vi "Cartesian_Experiment.vi"() -> ()   [LabVIEW 2016]
uses:
  <vilib>/gmath/NI_Gmath.lvlib
panel:
  out "Waveform Graph":dbl[][](graph)
  out "Action VIs":path[](array[path])=[path "C:/user/patrick/control_vi/Action_SubVIs/Set_B.vi", path "C:/user/patrick/control_vi/Action_SubVIs/Set_T.vi", path "C:/user/patrick/control_vi/Action_SubVIs/Set_Vsg1.vi", path "C:/user/patrick/control_vi/Action_SubVIs/Set_Vsg2.vi"]
  in  "Number of switch settings":i32
  in  "Tab Control":T1(tab)=enum."File Settings"
  in  "Scan Array (Slow to Fast: priority = 0 to N)":T2(array[cluster])=[{"Ramp Cluster"={"Max"=0.0, "Min"=0.0, "step size"=0.004, "cycles (1,2,...)"=0, "phase (deg)"=0.0, "function (ramp)"=enum."Ramp"}, "Priority"=0, "Action"=0, "Action 2"=0}, {"Ramp Cluster"={"Max"=0.15, "Min"=-0.08, "step size"=0.01, "cycles (1,2,...)"=0, "phase (deg)"=0.0, "function (ramp)"=enum."Ramp"}, "Priority"=2, "Action"=0, "Action 2"=0}, {"Ramp Cluster"={"Max"=0.15, "Min"=-0.15, "step size"=0.001, "cycles (1,2,...)"=0, "phase (deg)"=0.001, "function (ramp)"=enum."Ramp"}, "Priority"=1, "Action"=0, "Action 2"=0}] {"Action 2" items=["single value", "ramp", "vector ramp", "other..."]; "Action" items=["Set_B", "Set_T", "Set_Vsg1", "Set_Vsg2"]; "Ramp Cluster"."phase (deg)" format="%#.4p"; "Ramp Cluster"."cycles (1,2,...)" min=1; "Ramp Cluster"."step size" format="%#.4p"; "Ramp Cluster"."Min" format="%#_6p"; "Ramp Cluster"."Max" format="%#_6p"}
  in  "stop":bool
  in  "AVS_CalFolder":path=path "E:/Dropbox/Labview/LC Software/All Calibrations" caption="Action subVIs files path"
  in  "read T?":bool
  # "Ramp function: Min=START, Max=END\n\nOther functions: \nMax > Min, change phase to control starting value"
  # "Ao1 has a large offset (600mV), an offset it is hard wired to Vsg2"
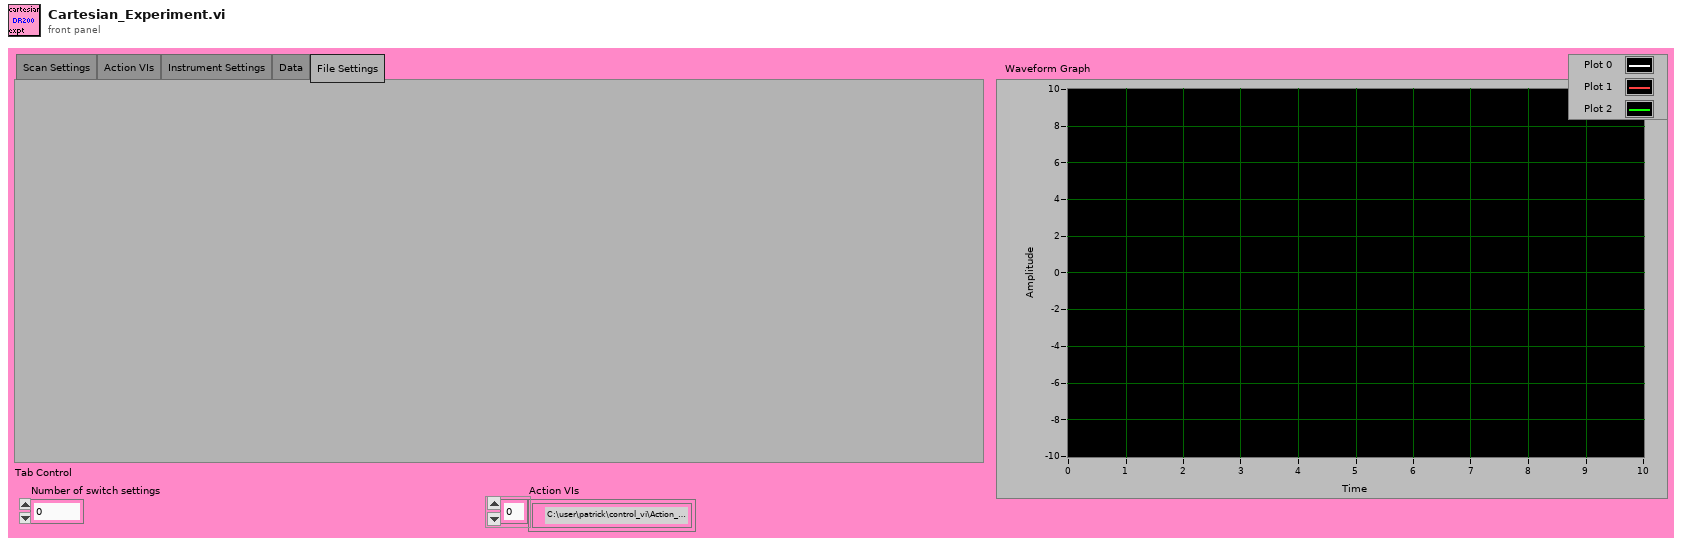
[diagram p1: front panel]
types:
  T1 = enum32{"Scan Settings", "Action VIs", "Instrument Settings", "Data", "File Settings"}
  T2 = cluster{"Ramp Cluster":cluster{"Max":dbl, "Min":dbl, "step size":dbl, "cycles (1,2,...)":i32, "phase (deg)":dbl, "function (ramp)":enum16{"Ramp", "Triangle", "Sine"}}, "Priority":i32, "Action":u16, "Action 2":u16}[]
  T3 = cluster{"Ramp Cluster":cluster{"Max":dbl, "Min":dbl, "step size":dbl, "cycles (1,2,...)":i32, "phase (deg)":dbl, "function (ramp)":enum16{"Ramp", "Triangle", "Sine"}}, "Priority":i32, "Action":u16, "Action 2":u16}
  T4 = enum16{"set T", "set B", "set Vsg1", "set Vsg2", "set lockin DC offset", "Switch"}
  T5 = cluster{"Max":dbl, "Min":dbl, "step size":dbl, "cycles (1,2,...)":i32, "phase (deg)":dbl, "function (ramp)":enum16{"Ramp", "Triangle", "Sine"}}
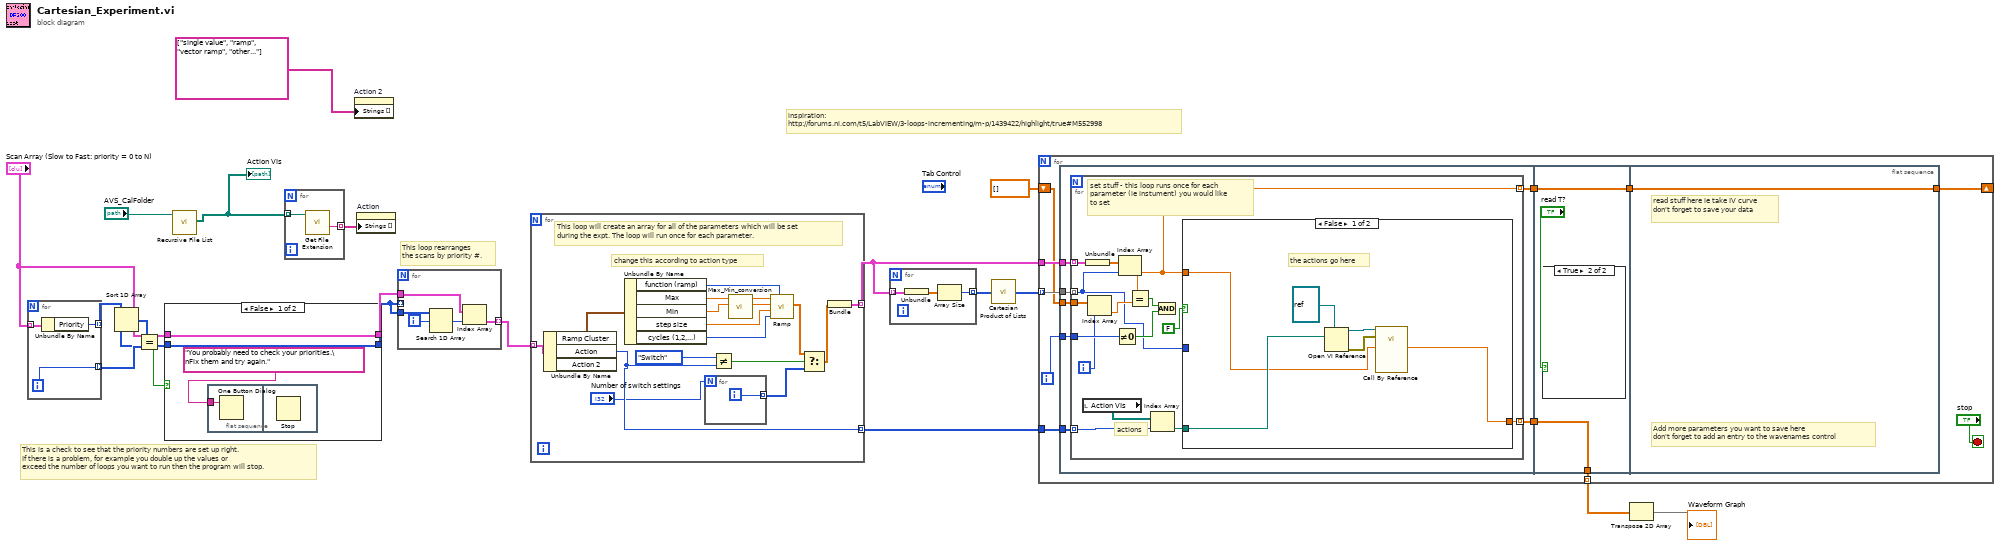
[diagram p0: block diagram]
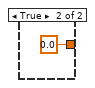
[diagram p2: hidden frame]
diagram:
  # "This loop rearranges\nthe scans by priority #."
  # "This is a check to see that the priority numbers are set up right. \nIf there is a problem, for example you double up the values or \nexceed the number of loops you want to run then the program will stop."
  # "inspiration:\nhttp://forums.ni.com/t5/LabVIEW/3-loops-incrementing/m-p/1439422/highlight/true#M552998"
  n1 = for {
    tunnel: "Scan Array (Slow to Fast: priority = 0 to N)" -> [w22] mode=indexing
    tunnel: [w21] -> w11 mode=indexing
    tunnel: [w20] -> w15 mode=indexing
    i -> [w20]
    n2 = Unbundle By Name(w22) -> ("Priority"=w21:i32)
  }
  n3 = Sort 1D Array(array=w11) -> (sorted array=w16:i32[])
  n4 = Equal?(x=w16, y=w15) -> (x = y?=w14:bool)
  n5 = case shown="False" w14 {
    tunnel: [w24 w28] -> w13
    tunnel: "Scan Array (Slow to Fast: priority = 0 to N)" -> [w24 w28]
    tunnel: [w25 w27] -> w10
    tunnel: w11 -> [w25 w27]
    frame False {
      n6 = flat-sequence {
        tunnel: "You probably need to check your priorities.\nFix them and try again." ("message") -> [w26]
        frame #0 {
          n7 = One Button Dialog(message=w26) -> ()  [unwired: 1 in, 1 out]
        }
        frame #1 {
          n8 = Stop() -> ()  [unwired: 1 in]
        }
      }
    }
    frame True {
    }
  }
  n9 = call <vilib>:"Recursive File List.vi"("Folder Path"="AVS_CalFolder") -> ("All Files in Dir"=w4:path[])  [unwired: 6 in, 4 out]
  "Action VIs" <- w4
  n10 = for {
    tunnel: w4 -> [w30] mode=indexing
    tunnel: [w29] -> w5 mode=indexing
    n11 = call <vilib>:"Get File Extension.vi"("file"=w30) -> ("filename without extension"=w29:string)  [unwired: 6 in, 4 out]
  }
  n12 = property on="Action 2" class="Ring (strict)"("Strings []"=string[] ["single value", "ramp", "vector ramp", "other..."]) -> ()  [unwired: 2 in, 2 out]
  n13 = property on="Action" class="Ring (strict)"("Strings []"=w5) -> ()  [unwired: 2 in, 2 out]
  n14 = for {
    tunnel: w13 -> [w35]
    tunnel: w10 -> [_] mode=indexing
    tunnel: [w34] -> w17 mode=indexing
    tunnel: w10 -> [w33]
    i -> [w32]
    n15 = Search 1D Array(1D array=w33, element=w32) -> (index of element=w31:i32)  [unwired: 1 in]
    n16 = Index Array(array=w35, index=w31) -> (element=w34:T3)
  }
  n17 = for {
    tunnel: [w51] -> w18 mode=indexing
    tunnel: w17 -> [w52] mode=indexing
    tunnel: [w41] -> w19 mode=indexing
    # "change this according to action type"
    # "This loop will create an array for all of the parameters which will be set\nduring the expt. The loop will run once for each parameter."
    n18 = Unbundle By Name(w52) -> ("Ramp Cluster"=w49:T5, "Action"=w41:u16)  [unwired: 1 out]
    n19 = Unbundle By Name(w49) -> ("function (ramp)"=w48:enum16{"Ramp", "Triangle", "Sine"}, "Max"=w47:dbl, "Min"=w46:dbl, "step size"=w44:dbl, "cycles (1,2,...)"=w43:i32)
    n20 = for {
      N: "Number of switch settings" -> [_]
      tunnel: [w53] -> w42 mode=indexing
      i -> [w53]
    }
    n21 = Not Equal?(x=T4."Switch" ("Action"), y=w41) -> (x != y?=w39:bool)
    n22 = call "Max_Min_conversion.vi"("Min"=w46, "Max"=w47) -> ("offset"=w45:dbl, "Amplitude"=w50:dbl)  [unwired: 8 in]
    n23 = call "Ramp.vi"("function (ramp)"=w48, "cycles (1,2,...)"=w43, "step size"=w44, "offset"=w45, "amplitude"=w50) -> ("Waveform Graph"=w38:dbl[])  [unwired: 4 in, 2 out]
    n24 = Select(t=w38, s=w39, f=w42) -> (s? t:f=w37:dbl[])
    n25 = Bundle("Waveform Graph"=w37) -> (w51:cluster{"Waveform Graph":dbl[]})  [unwired: 1 in]
  }
  n26 = for {
    tunnel: w18 -> [w56] mode=indexing
    tunnel: [w54] -> w9 mode=indexing
    n27 = Unbundle(w56) -> ("Waveform Graph"=w55:dbl[])
    n28 = Array Size(array=w55) -> (size(s)=w54:i32)
  }
  n29 = call <vilib>:"Cartesian Product of Lists.vi"("Number of Elements in Each List"=w9) -> ("Cartesian Product of Lists"=w7:i32[][])
  n30 = for {
    tunnel: w7 -> [w67] mode=indexing
    tunnel: w18 -> [w66]
    tunnel: w19 -> [w65]
    shift-right: [w64] -> _
    shift-left: dbl[] [] -> [w63]
    tunnel: [w57] -> w3 mode=indexing
    i -> [w59]
    stop <- "stop" stop-if-true
    n31 = flat-sequence {
      tunnel: w67 -> [w74]
      tunnel: w66 -> [w73]
      tunnel: w65 -> [w72]
      tunnel: w63 -> [w70]
      tunnel: w59 -> [w69]
      tunnel: [w71] -> w62
      tunnel: [w68] -> w58
      tunnel: w62 -> [w99]
      tunnel: [w99] -> w61
      tunnel: w58 -> [w97]
      tunnel: [w97] -> w57
      tunnel: w61 -> [w100]
      tunnel: [w100] -> w64
      frame #0 {
        n32 = for {
          tunnel: w74 -> [w80] mode=indexing
          tunnel: w73 -> [w89] mode=indexing
          tunnel: w72 -> [w79] mode=indexing
          tunnel: [w87] -> w71 mode=indexing
          tunnel: w70 -> [w84]
          tunnel: w69 -> [w82]
          tunnel: [w76] -> w68 mode=indexing
          i -> [w81]
          # "actions"
          # "set stuff - this loop runs once for each\nparameter (ie instument) you would like\nto set"
          n33 = local read "Action VIs"() -> (w78:path[])
          n34 = Unbundle(w89) -> ("Waveform Graph"=w88:dbl[])
          n35 = Index Array(array=w84, index=w81) -> (element=w83:dbl)
          n36 = Not Equal To 0?(x=w82) -> (x != 0?=w86:bool)
          n37 = Index Array(array=w88, index=w80) -> (element=w87:dbl)
          n38 = Equal?(x=w87, y=w83) -> (x = y?=w85:bool)
          n39 = Index Array(array=w78, index=w79) -> (element=w77:path)
          n40 = And(x=w85, y=w86) -> ()  [unwired: 1 out]
          n41 = case shown="False" FALSE {
            tunnel: w87 -> [w91 _]
            tunnel: w80 -> [_ _]
            tunnel: w77 -> [w92 _]
            tunnel: [w90 0.0 ("Numeric 2")] -> w76
            frame False {
              # "the actions go here"
              n42 = Open VI Reference(type specifier VI Refnum (for type only)=refnum<vi> refnum, vi path=w92) -> (vi reference=w93:refnum<vi>, error out=w94:errorcluster)  [unwired: 4 in]
              n43 = call-by-ref "?"(reference=w93, error in=w94, "Numeric"=w91) -> ("Numeric 2"=w90:dbl)  [unwired: 6 in, 2 out]
            }
            frame True {
            }
          }
        }
      }
      frame #1 {
        n44 = case shown="True" "read T?" {
          frame False {
          }
          frame True {
          }
        }
      }
      frame #2 {
        # "Add more parameters you want to save here\ndon't forget to add an entry to the wavenames control"
        # "read stuff here ie take IV curve\ndon't forget to save your data"
      }
    }
  }
  n45 = Transpose 2D Array(2D array=w3) -> (transposed array=→"Waveform Graph":dbl[][])
